vi "Get Image Timings.vi"(8 "error in (no error)":errorcluster, 11 "Save Image in":refnum<class "Save Image.lvclass">) -> (0 "error out":errorcluster, 3 "Save Image out":refnum<class "Save Image.lvclass">)   [LabVIEW 2018, in "Save Image.lvclass"]
uses:
  Save Image.lvclass
  Save Image.lvclass/Save Image.ctl
  Header/Header.lvclass
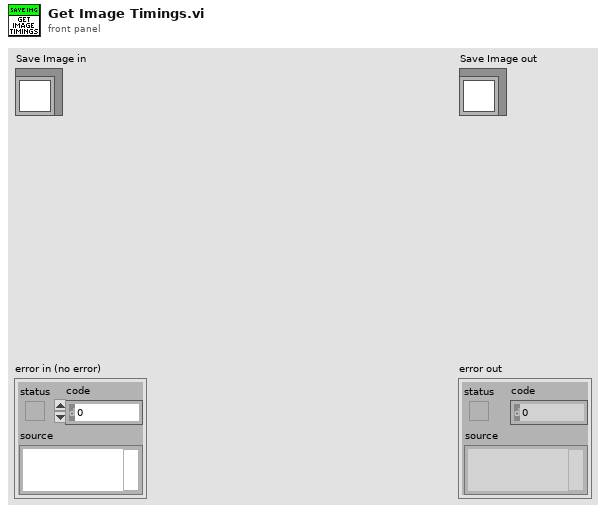
[diagram p1: front panel]
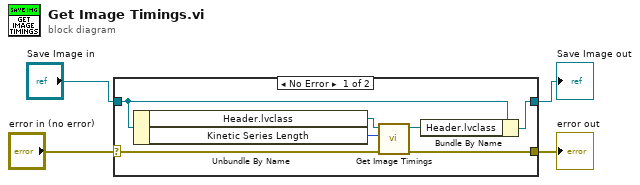
[diagram p0: block diagram]
diagram:
  n1 = case shown="No Error" "error in (no error)" {
    selector: "error in (no error)" -> [w6 w13]
    tunnel: [w5 w13] -> w3
    tunnel: [w10 w12] -> w1
    tunnel: "Save Image in" -> [w11 w12]
    frame No Error {
      n2 = Unbundle By Name(w11) -> ("Header.lvclass"=w9:refnum<class "Header.lvclass">, "Kinetic Series Length"=w7:u16)
      n3 = call "Get Image Timings.vi"("error in (no error)"=w6, "Kinetic Series Lenght"=w7, "Header in"=w9) -> ("error out"=w5:errorcluster, "Header out"=w8:refnum<class "Header.lvclass">)  [unwired: 7 in]
      n4 = Bundle By Name(cluster=w11, "Header.lvclass"=w8) -> (w10:refnum<class "Save Image.lvclass">)
    }
    frame Error {
    }
  }
  "error out" <- w3
  "Save Image out" <- w1
